vi "CheckConnect.vi"(8 "error in (no error)":errorcluster, 11 "BaseDriver in":refnum<class "BaseDriver.lvclass">) -> (0 "error out":errorcluster, 3 "BaseDriver out":refnum<class "BaseDriver.lvclass">)   [LabVIEW 2013, in "BaseDriver.lvclass"]
doc: "Checks if the Reader is still connected. If not, emits a \"Connection lost\" response"
uses:
  BaseDriver.lvclass
  BaseDriver.lvclass/BaseDriver.ctl
  Reader/BaseReader/BaseReader.lvclass
  driver_status.ctl
  response.ctl
  Responder/BaseResponder/BaseResponder.lvclass
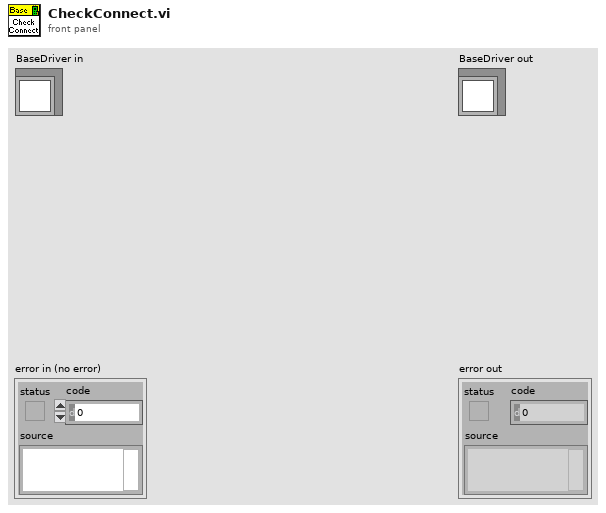
[diagram p1: front panel]
types:
  T1 = typedef "response.ctl" = cluster{"driver status":T2, "Sender":string, "Type":i32, "Variant":variant}
  T2 = typedef "driver_status.ctl" = enum16{"Normal", "Startup", "Connection lost", "Reconnected", "Timeout", "Idle", "Busy"}
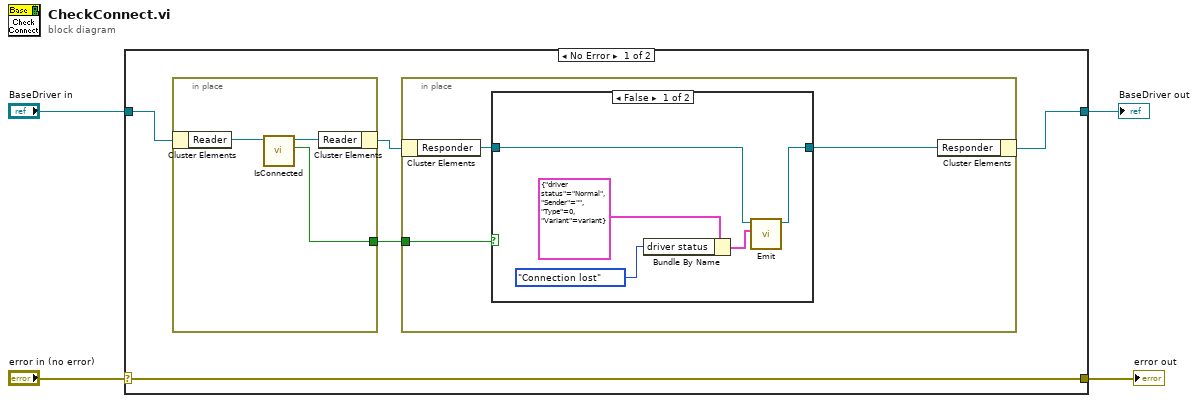
[diagram p0: block diagram]
diagram:
  n1 = case shown="No Error" "error in (no error)" {
    selector: "error in (no error)" -> [w9 w23]
    tunnel: [w9 w23] -> w3
    tunnel: [w5 w22] -> w1
    tunnel: "BaseDriver in" -> [w8 w22]
    frame No Error {
      n2 = in-place "In Place Element Structure" {
        in-place-border: [w20] -> w6
        n3 = in-place-cluster #1(w8) -> ("Reader"=w19:refnum<class "BaseReader.lvclass">)
        n4 = call-dynamic "IsConnected.vi"("BaseReader in"=w19) -> ("connected?"=w20:bool, "BaseReader out"=w21:refnum<class "BaseReader.lvclass">)  [unwired: 8 in, 1 out]
        n5 = in-place-cluster #1("Reader"=w21) -> (w7:refnum<class "BaseDriver.lvclass">)
      }
      n6 = in-place "In Place Element Structure" {
        in-place-border: w6 -> [w11]
        n7 = in-place-cluster #2(w7) -> ("Responder"=w10:refnum<class "BaseResponder.lvclass">)
        n8 = case shown="False" w11 {
          tunnel: w10 -> [w17 w18]
          tunnel: [w16 w18] -> w12
          frame False {
            n9 = Bundle By Name(cluster=T1 {"driver status"=enum."Normal", "Sender"="", "Type"=0, "Variant"=variant} ("response"), "driver status"=driver_status."Connection lost") -> (w14:T1)
            n10 = call-dynamic "Emit.vi"("response"=w14, "BaseResponder in"=w17) -> ("BaseResponder out"=w16:refnum<class "BaseResponder.lvclass">)  [unwired: 8 in, 1 out]
          }
          frame True {
          }
        }
        n11 = in-place-cluster #2("Responder"=w12) -> (w5:refnum<class "BaseDriver.lvclass">)
      }
    }
    frame Error {
    }
  }
  "error out" <- w3
  "BaseDriver out" <- w1
